vi "Write_TCP_Serial (SubVI).vi"(8 "error in (no error)":errorcluster, 11 "connectionParamIn":T1={"ReadIntParam"=TRUE, "ReadDescrParam"=FALSE, "ReadFloatParam"=TRUE, "debug"=FALSE, "ReadJSON"=TRUE, "IP_address"="192.168.1.216", "N_attempts"=3, "type_con"=enum."TCP", "MB_address"=1, "VISA"="COM1", "connection ID"=refnum, "nameDevices"="", "timeout"=3000, "port"=2000, "type_version"="0F0C0001", "baud_rate"=115200, "VersionControl"=TRUE, "TCP_conn"=TRUE, "WindowSize"=700}) -> (0 "error out":errorcluster, 2 "data out":string, 3 "connectionParamOut":T1={"ReadIntParam"=TRUE, "ReadDescrParam"=FALSE, "ReadFloatParam"=TRUE, "debug"=FALSE, "ReadJSON"=TRUE, "IP_address"="192.168.1.216", "N_attempts"=3, "type_con"=enum."TCP", "MB_address"=1, "VISA"="COM1", "connection ID"=refnum, "nameDevices"="", "timeout"=3000, "port"=2000, "type_version"="0F0C0001", "baud_rate"=115200, "VersionControl"=TRUE, "TCP_conn"=TRUE, "WindowSize"=700})   [LabVIEW 2017, in "LV_Unicorn.lvlib"]
uses:
  LV_Unicorn.lvlib
  Control/unicorn_conn.ctl
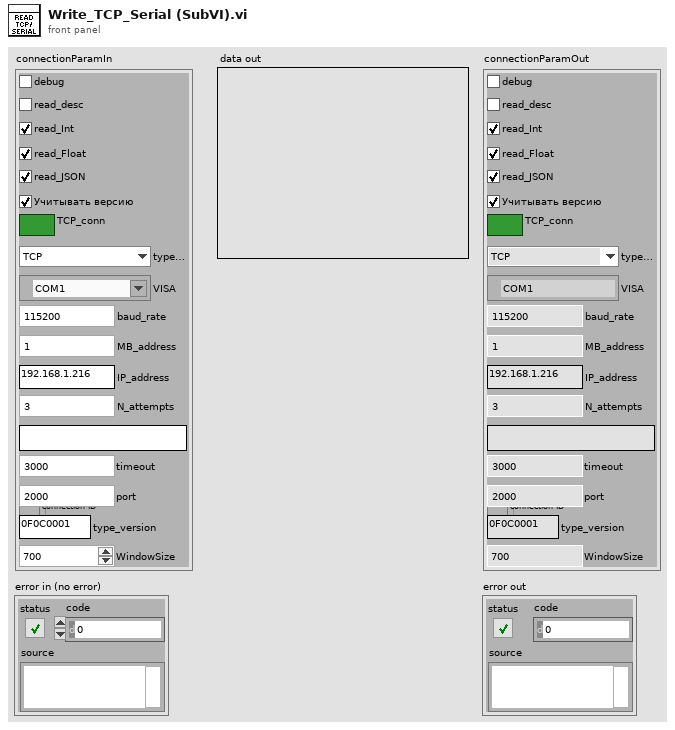
[diagram p1: front panel]
types:
  T1 = typedef "LV_Unicorn.lvlib/unicorn_conn.ctl" = cluster{"ReadIntParam":bool, "ReadDescrParam":bool, "ReadFloatParam":bool, "debug":bool, "ReadJSON":bool, "IP_address":string, "N_attempts":i32, "type_con":enum16{"Serial", "TCP"}, "MB_address":i32, "VISA":refnum<visa-resource-name>, "connection ID":refnum<k5>, "nameDevices":string, "timeout":i32, "port":u16, "type_version":string, "baud_rate":u32, "VersionControl":bool, "TCP_conn":bool, "WindowSize":i32}
  T2 = enum16{"Standard", "Buffered", "CRLF", "Immediate"}
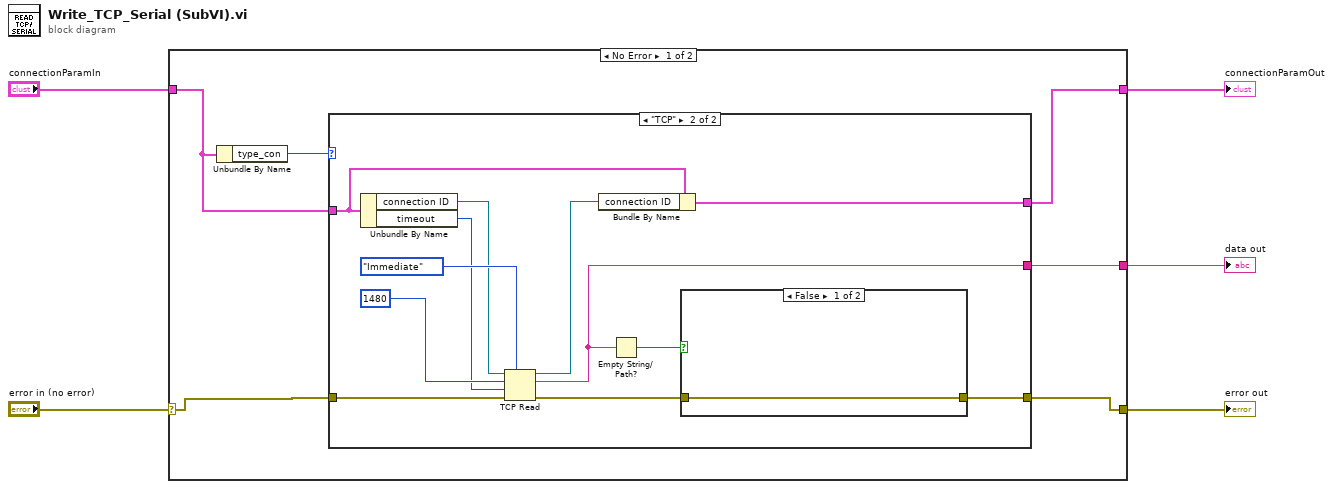
[diagram p0: block diagram]
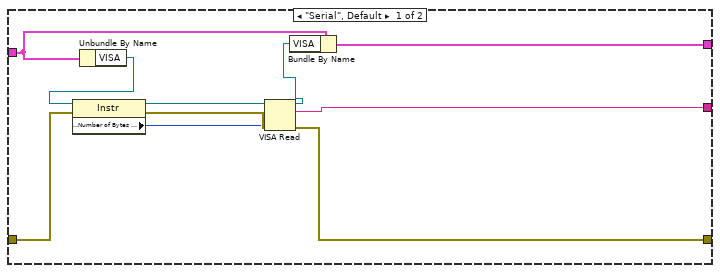
[diagram p2: hidden frame]
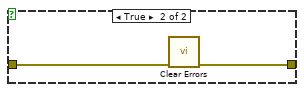
[diagram p3: hidden frame]
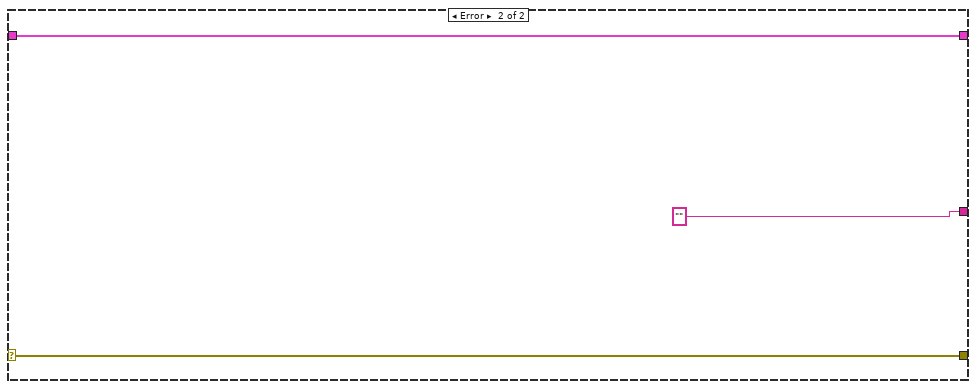
[diagram p4: hidden frame]
diagram:
  n1 = case shown="No Error" "error in (no error)" {
    selector: "error in (no error)" -> [w6 w39]
    tunnel: [w11 w39] -> w5
    tunnel: "connectionParamIn" -> [w9 w38]
    tunnel: [w8 w38] -> w3
    tunnel: [w7 "" ("data out")] -> w2
    frame No Error {
      n2 = Unbundle By Name(w9) -> ("type_con"=w10:enum16{"Serial", "TCP"})
      n3 = case shown="\"TCP\"" w10 {
        tunnel: w6 -> [w18 w33]
        tunnel: [w17 w25] -> w7
        tunnel: [w16 w23] -> w11
        tunnel: w9 -> [w14 w28]
        tunnel: [w12 w26] -> w8
        frame "Serial", Default {
          n4 = Unbundle By Name(w14) -> ("VISA"=w15:refnum<visa-resource-name>)
          n5 = property class="Instr"(reference=w15, error in=w18) -> (reference out=w20:refnum<visa-resource-name>, error out=w21:errorcluster, "Serial Settings:Number of Bytes at Serial Port"=w19:u32)
          n6 = VISA Read(VISA resource name=w20, byte count=w19, error in (no error)=w21) -> (VISA resource name out=w13:refnum<visa-resource-name>, read buffer=w17:string, error out=w16:errorcluster)  [unwired: 1 out]
          n7 = Bundle By Name(cluster=w14, "VISA"=w13) -> (w12:T1)
        }
        frame "TCP" {
          n8 = Unbundle By Name(w28) -> ("connection ID"=w30:refnum<k5>, "timeout"=w29:i32)
          n9 = TCP Read(connection ID=w30, bytes to read=1480, error in (no error)=w33, 7:T2."Immediate" ("mode (standard)"), 9:w29) -> (connection ID out=w27:refnum<k5>, data out=w25:string, error out=w22:errorcluster)
          n10 = Bundle By Name(cluster=w28, "connection ID"=w27) -> (w26:T1)
          n11 = Empty String/Path?(string/path=w25) -> (empty?=w24:bool)
          n12 = case shown="False" w24 {
            tunnel: [w34 w35] -> w23
            tunnel: w22 -> [w34 w36]
            frame False {
            }
            frame True {
              n13 = call <vilib>:"Clear Errors.vi"("error in (no error)"=w36) -> ("error out"=w35:errorcluster)  [unwired: 5 in, 1 out]
            }
          }
        }
      }
    }
    frame Error {
    }
  }
  "error out" <- w5
  "connectionParamOut" <- w3
  "data out" <- w2
